vi "RT_small.vi"() -> ()   [LabVIEW 2018]
uses:
  <vilib>/rvi/interface/nirviOpenFPGA/nirviOpenFPGA.xnode
  <vilib>/rvi/interface/nirviCloseFPGA/nirviCloseFPGA.xnode
  <vilib>/rvi/interface/nirviReadWriteControl/nirviReadWriteControl.xnode
  <vilib>/rvi/interface/Simulation/niFpgaSimulationCallBeginRW.vi
  <vilib>/rvi/errors/niLvFpgaAdjustHostInterfaceError.vi
  <vilib>/FPGAPlugInAG/Dynamic/niLvFpga_Close_Dynamic.vi
  NiFpgaLv.dll
  <vilib>/Utility/error.llb/Error Cluster From Error Code.vi
  <vilib>/addons/control/pid/NI_PID_pid.lvlib
  <vilib>/addons/control/pid/pid.llb/PID (DBL).vi
  FPGA Bitfiles/DQNcarpolelvsim_FPGATarget_FPGAsmall2_d4itNFSFwjs.lvbitx
  FPGA_small2.vi
  <vilib>/FPGAPlugInAG/myRIO-1900/niLvFpga_Open_myRIO-1900.vi
  <vilib>/rvi/interface/common/dynamic/niFpgaDynamicAddResources.vi
panel:
  out "gap_pos":i16
  in  "setpoint":dbl format="%.2f"
  out "states":dbl[](array[numeric])
  out "busy":bool
  out "off_track":bool
  out "output":dbl=559.250913333665 format="%.2f"
  in  "output range":cluster{"output high":dbl, "output low":dbl}={"output high"=700.0, "output low"=550.0} {"output low" format="%.2f"; "output high" format="%.2f"}
  in  "dt (s)":dbl=0.001 format="%.3f"
  in  "PID gains":T1={"proportional gain (Kc)"=0.0005, "integral time (Ti, min)"=0.001, "derivative time (Td, min)"=0.001} {"derivative time (Td, min)" format="%.5f"; "integral time (Ti, min)" format="%.5f"; "proportional gain (Kc)" format="%.4f"}
  out "speed Chart":i16(graph)
  out "position":i16=209
  in  "stop":bool
  in  "set_point":i16(slide)=207 scale=-800.0..800.0
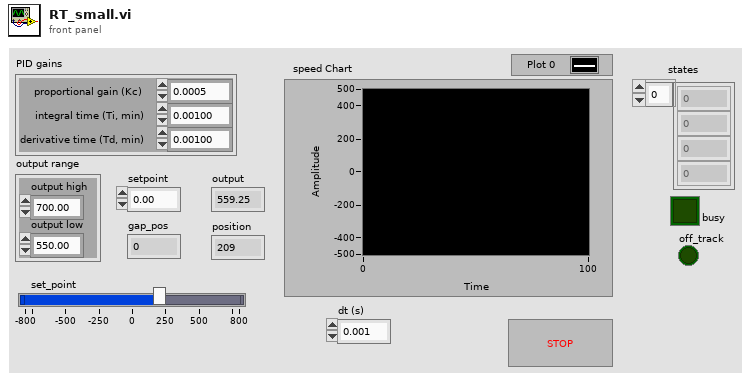
[diagram p1: front panel]
types:
  T1 = cluster{"proportional gain (Kc)":dbl, "integral time (Ti, min)":dbl, "derivative time (Td, min)":dbl}
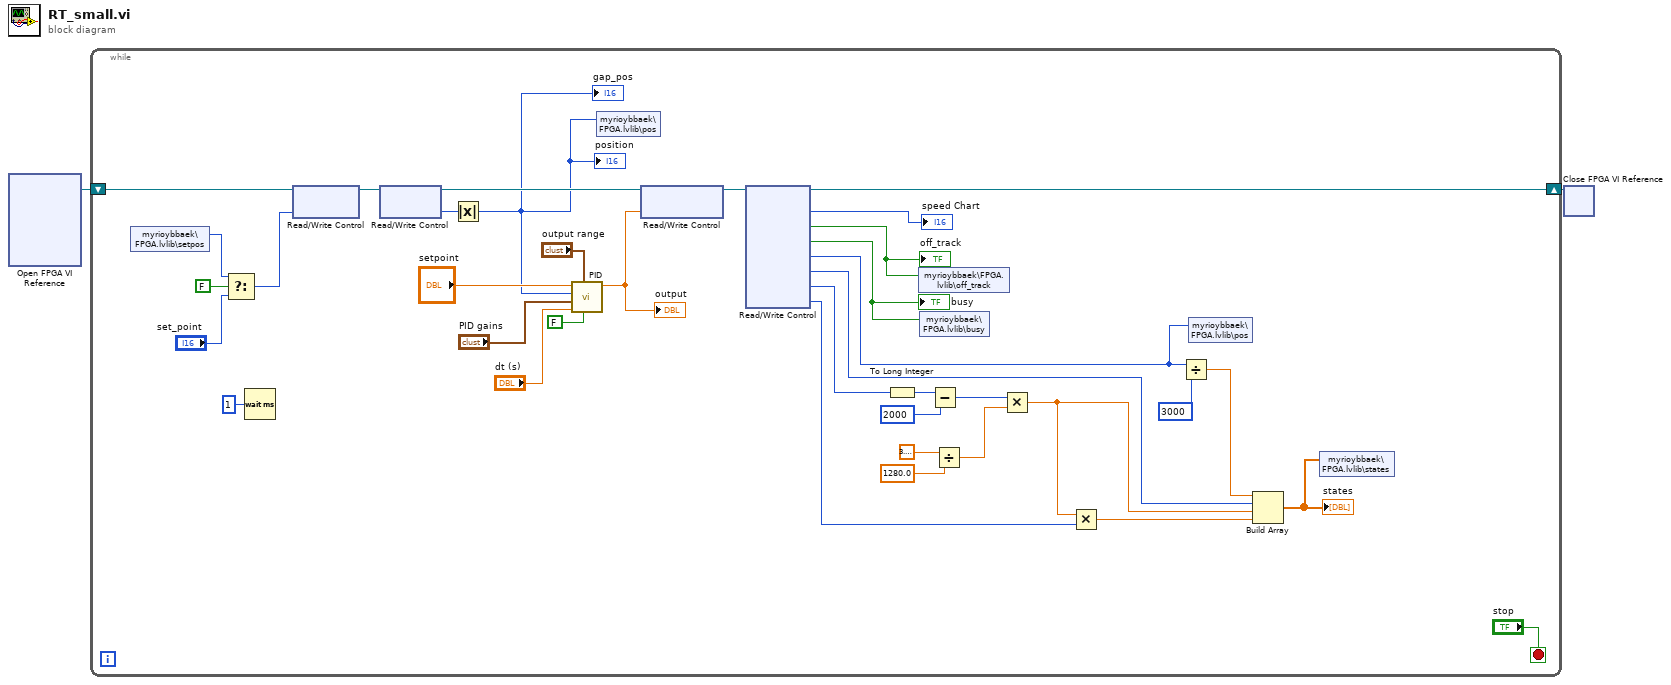
[diagram p0: block diagram]
diagram:
  n1 = xnode "Open FPGA VI Reference"() -> ("FPGA VI Reference Out"=w2:refnum<k20>)  [unwired: 2 in, 1 out]
  n2 = while {
    shift-right: [w27] -> w1
    shift-left: w2 -> [w39]
    stop <- "stop" stop-if-true
    n3 = shared-variable "myrioybbaek\\FPGA.lvlib\\setpos"() -> (w24:i16)  [unwired: 1 in, 1 out]
    n4 = Select(t=w24, s=FALSE, f="set_point") -> (s? t:f=w23:i16)
    n5 = Wait (ms)(milliseconds to wait=u32 1) -> ()  [unwired: 1 out]
    n6 = xnode "Read/Write Control"("FPGA VI Reference In"=w39, "set_point"=w23) -> ("FPGA VI Reference Out"=w36:refnum<k20>)  [unwired: 1 in, 1 out]
    n7 = xnode "Read/Write Control"("FPGA VI Reference In"=w36) -> ("FPGA VI Reference Out"=w31:refnum<k20>, "position"=w26:i16)  [unwired: 1 in, 1 out]
    n8 = Absolute Value(x=w26) -> (abs(x)=w3:i16)
    "position" <- w3
    "gap_pos" <- w3
    n9 = call-poly <vilib>:"PID.vi"("reinitialize? (F)"=FALSE, "output range"="output range", "dt (s)"="dt (s)", "PID gains"="PID gains", "process variable"=w3, "setpoint"="setpoint") -> ("output"=w32:dbl)  [unwired: 4 in, 1 out]
    "output" <- w32
    n10 = shared-variable "myrioybbaek\\FPGA.lvlib\\pos"(w3) -> ()  [unwired: 1 in, 1 out]
    n11 = xnode "Read/Write Control"("FPGA VI Reference In"=w31, "dt_pwm_ms"=w32) -> ("FPGA VI Reference Out"=w30:refnum<k20>)  [unwired: 1 in, 1 out]
    n12 = xnode "Read/Write Control"("FPGA VI Reference In"=w30) -> ("FPGA VI Reference Out"=w27:refnum<k20>, "speed"=→"speed Chart":i16, "off_track"=w21:bool, "busy"=w8:bool, "position"=w9:i16, "speed"=w6:i16, "AI0"=w7:u16, "dAI"=w5:i16)  [unwired: 1 in, 1 out]
    "off_track" <- w21
    "busy" <- w8
    n13 = To Long Integer(number=w7) -> (32bit integer=w20:i32)
    n14 = shared-variable "myrioybbaek\\FPGA.lvlib\\off_track"(w21) -> ()  [unwired: 1 in, 1 out]
    n15 = shared-variable "myrioybbaek\\FPGA.lvlib\\busy"(w8) -> ()  [unwired: 1 in, 1 out]
    n16 = Subtract(x=w20, y=u16 2000) -> (x-y=w18:i32)
    n17 = Divide(x=3.141592653589793, y=1280.0) -> (x/y=w19:dbl)
    n18 = Multiply(x=w18, y=w19) -> (x*y=w16:dbl)
    n19 = Multiply(x=w16, y=w5) -> (x*y=w17:dbl)
    n20 = Divide(x=w9, y=i16 3000) -> (x/y=w12:dbl)
    n21 = shared-variable "myrioybbaek\\FPGA.lvlib\\pos"(w9) -> ()  [unwired: 1 in, 1 out]
    n22 = Build Array(w12, w6, w16, w17) -> (w10:dbl[])
    "states" <- w10
    n23 = shared-variable "myrioybbaek\\FPGA.lvlib\\states"(w10) -> ()  [unwired: 1 in, 1 out]
  }
  n24 = xnode "Close FPGA VI Reference"("FPGA VI Reference In"=w1) -> ()  [unwired: 1 in, 1 out]
